vi "CMD Only (RT).vi"() -> ()   [LabVIEW 2013]
uses:
  Type Defs/Controller Names.ctl
  Type Defs/Sequence States.ctl
  Type Defs/CAN Mode.ctl
  Type Defs/Controller List.ctl
  <vilib>/FPGAPlugInAG/sbRIO-9626/niLvFpga_Open_sbRIO-9626.vi
  <vilib>/rvi/interface/common/dynamic/niFpgaDynamicAddResources.vi
  <vilib>/FPGAPlugInAG/Dynamic/niLvFpga_Reset_Dynamic.vi
  <vilib>/rvi/interface/common/niFpgaWaitOnOcc.vi
  <vilib>/Utility/error.llb/Error Cluster From Error Code.vi
  <vilib>/rvi/errors/niLvFpgaAdjustHostInterfaceError.vi
  <vilib>/FPGAPlugInAG/Dynamic/niLvFpga_Run_Dynamic.vi
  <vilib>/rvi/interface/nirviOpenFPGA/nirviOpenFPGA.xnode
  FPGA Bitfiles/CMD Only.lvbitx
  <vilib>/rvi/interface/nirviMethod/nirviMethod.xnode
  <vilib>/rvi/interface/nirviReadWriteControl/nirviReadWriteControl.xnode
  NiFpgaLv.dll
  <vilib>/rvi/interface/Simulation/niFpgaSimulationCallBeginRW.vi
  <vilib>/NI_Real-Time Target Support.lvlib
panel:
  in  "Monitoring Tab":enum32{"Page 1", "Page 2"}(tab)
  in  "Command":dbl min=10.0 max=100.0 step=0.1 format="%#.2f"
  in  "pb.Zero CMDs":bool
  out "CPU Usage:":dbl=7.74131899555212 format="%.1f"
  in  "Controller Type:":T1
  in  "Title":string="TI Automotive sbRIO, v2.1"
  out "CAN CMD":dbl
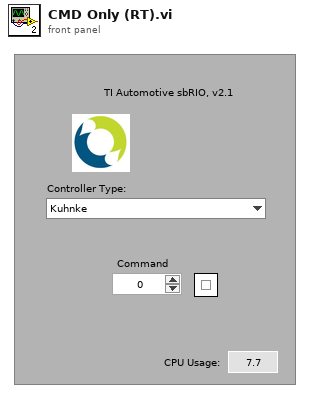
[diagram p1: front panel]
types:
  T1 = typedef "Controller Names.ctl" = enum16{"Kuhnke", "Conti", "Helbako", "TI PWM", "PSA", "Hella Gas", "Hella Diesel", "8 Comm", "10 Comm", "8 Comm Hella", "10 Comm Hella", "8 Comm Omron", "10 Comm Omron", "8 Comm Nissan", "10 Comm Nissan"}
  T2 = cluster{"Controller Name":T1, "CommSeg":i32, "PWM?":bool, "Frequency":i32, "Low Command":dbl, "High Command":dbl, "Stop Command":dbl, "Command Step":dbl, "Solenoid Stop?":bool, "Controller?":bool}
  T3 = typedef "CAN Mode.ctl" = enum16{"Init", "Read", "Write", "Close"}
  T4 = typedef "Sequence States.ctl" = enum16{"Main", "Init Files", "Init", "Save As", "Start Profile", "Check Step Time", "Restarts Alarm", "Run Step", "Stop Profile", "Cycle Reset", "Time Reset", "Time Reset All", "Time Set", "Tare CTs", "Save Profile", "Open Profile", "Get Profiles", "Update Screen", "Save Status", "Set Manual CMD", "Reset Restarts", "Reset Total Restarts", "Reset Cogs", "Disable Background", "Enable Background", "Get/Release Control", "Init AKLH", "Save AKLH", "Log Fuel Change", "Update Data Stream", "Init TenHz", "Read TenHz", "Remote Timer Reset", "Record Frequency Change", "Controller Change"}
  T5 = cluster{"Last Update":dbl, "Update Screen":bool, "Command":dbl, "Client?":bool, "Update Profile":bool, "Login":bool, "Stop Cmd":dbl, "Controller":cluster{"Controller Name":T1, "CommSeg":i32, "PWM?":bool, "Frequency":i32, "Low Command":dbl, "High Command":dbl, "Stop Command":dbl, "Command Step":dbl, "Solenoid Stop?":bool, "Controller?":bool}, "Controller Type:":T1}
  T6 = typedef "Controller List.ctl" = cluster{"Controller Name":T1, "CommSeg":i32, "PWM?":bool, "Frequency":i32, "Low Command":dbl, "High Command":dbl, "Stop Command":dbl, "Command Step":dbl, "Solenoid Stop?":bool, "Controller?":bool}[]
  T7 = typedef "LVRemotePanelConnectionsTypeDef.ctl" = cluster{"VI Name":string, "Remote":string, "UserName":string, "Port":i32, "Status":enum32{"Viewing", "Waiting For Control", "Controlling"}, "Create Time":timestamp, "Status Time":timestamp, "Control End Time":timestamp}[]
  T8 = typedef "NI_Real-Time Target Support.lvlib/RT CPU Load.ctl" = cluster{"Total (%)":dbl, "Time Critical (%)":dbl, "Timed Structures (%)":dbl, "High (%)":dbl, "Above Normal (%)":dbl, "Normal (%)":dbl, "Background (%)":dbl, "Idle (%)":dbl, "ISR (%)":dbl}
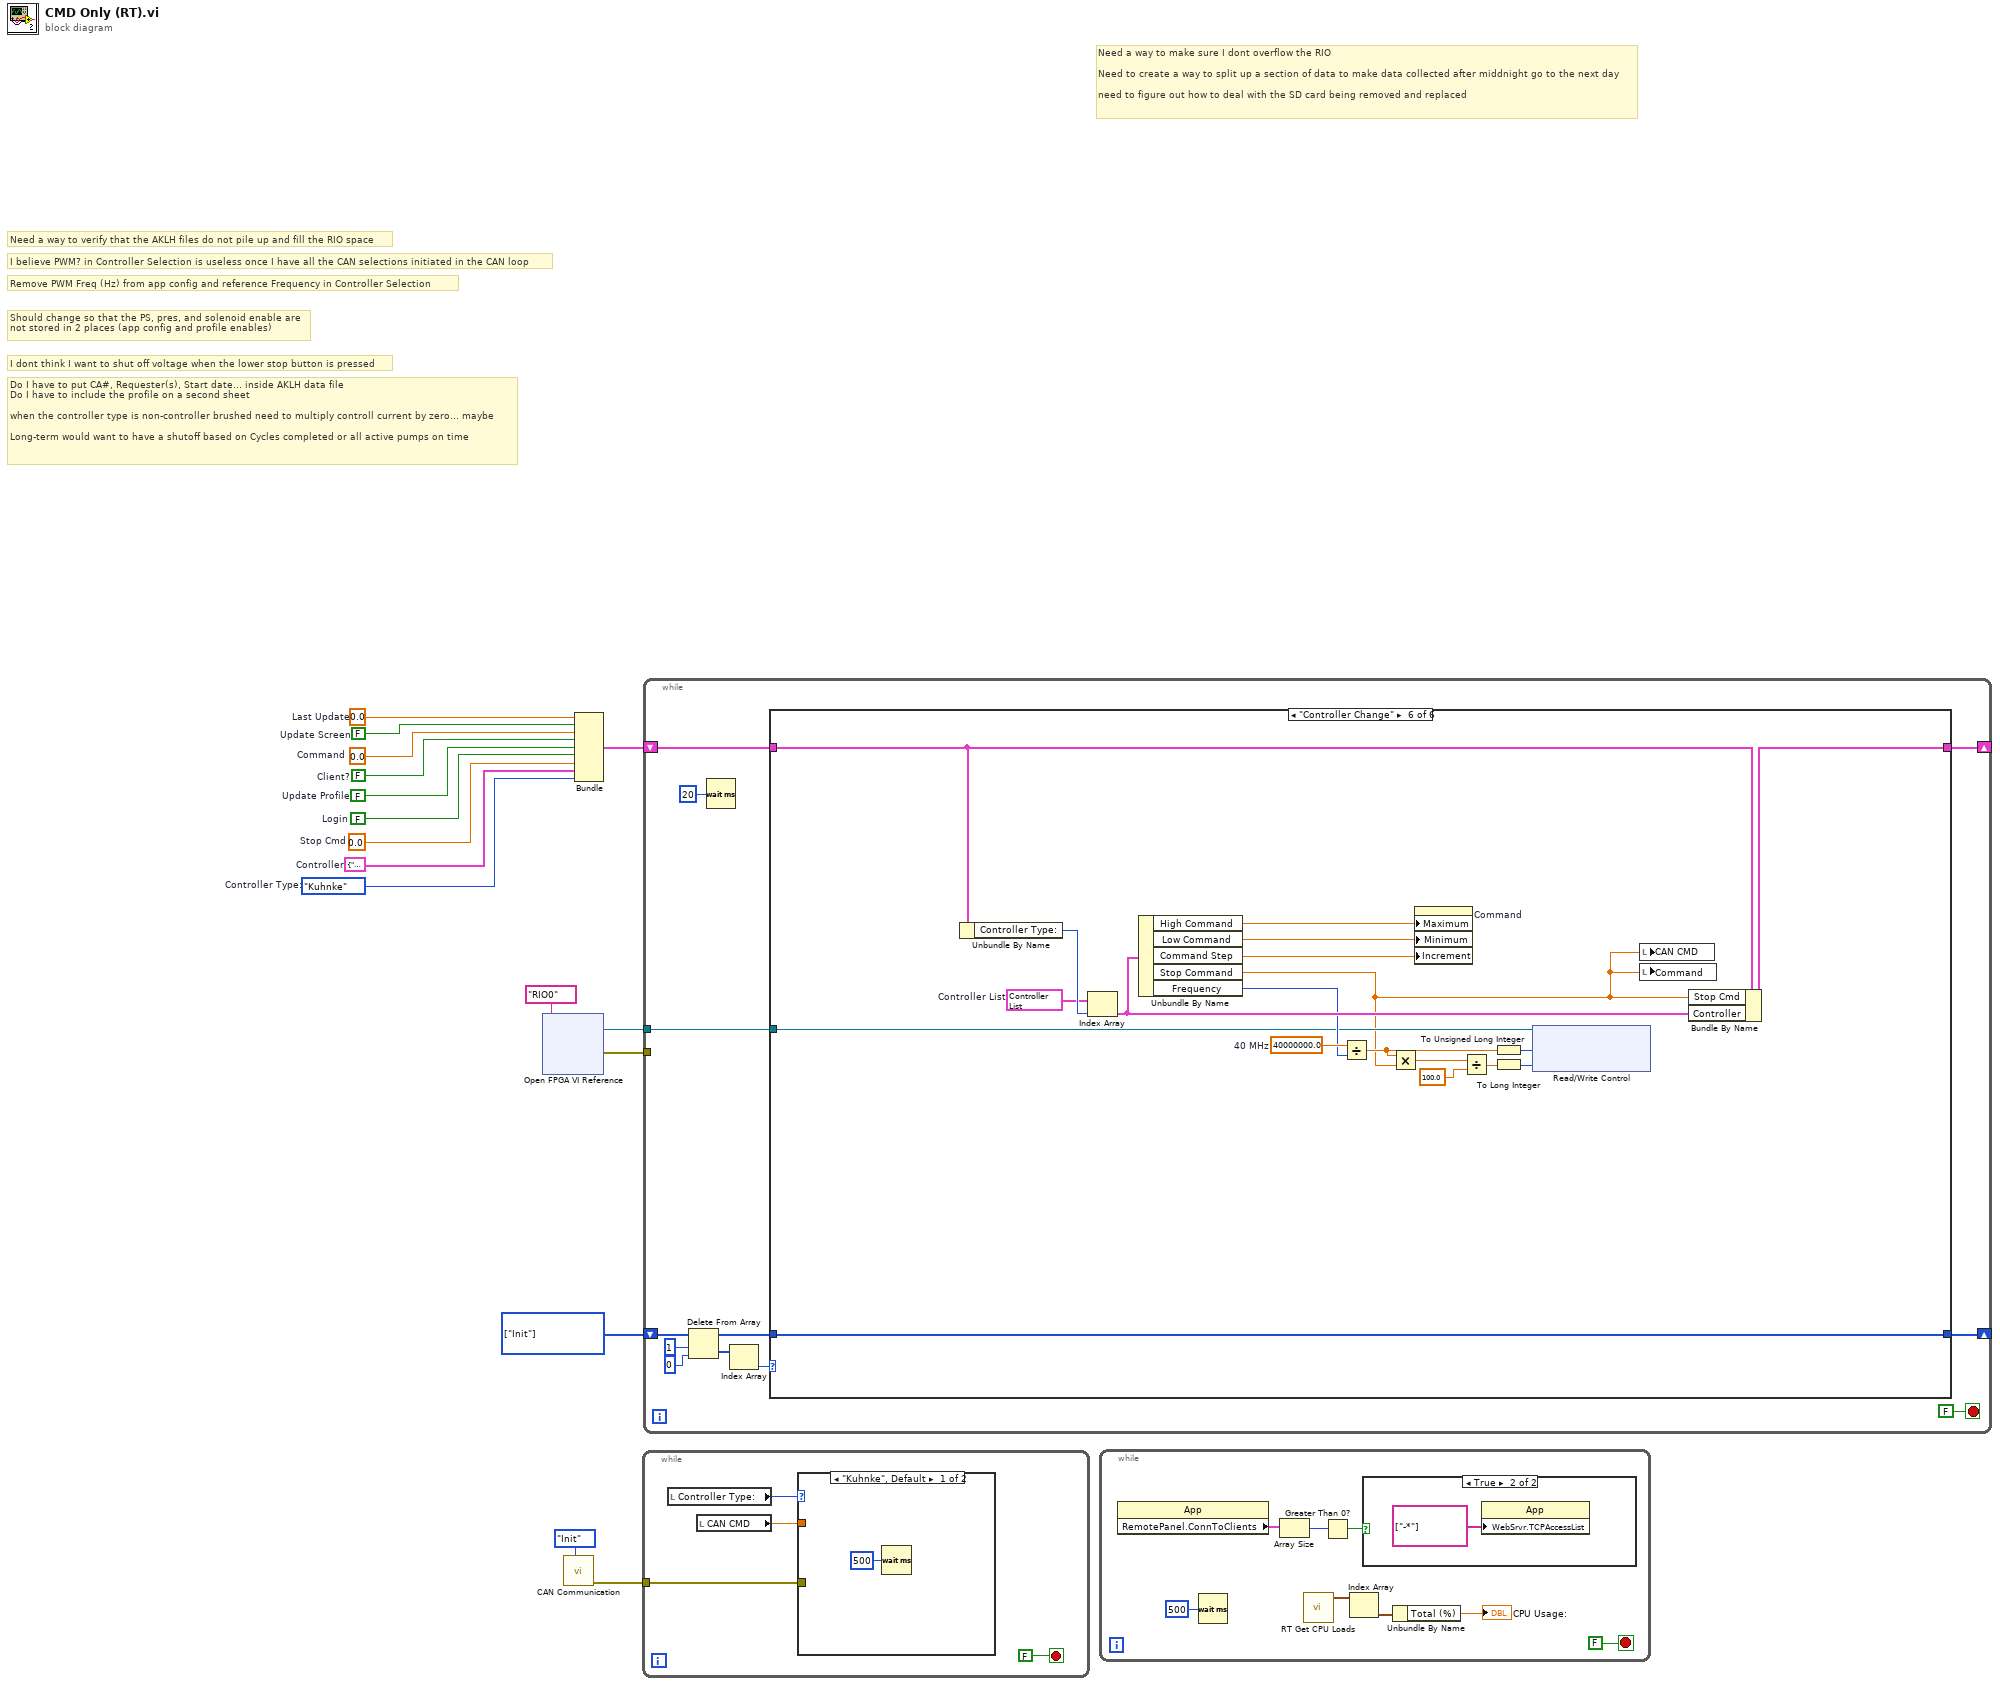
[diagram p0: block diagram]
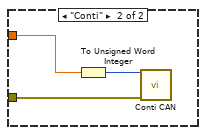
[diagram p2: hidden frame]
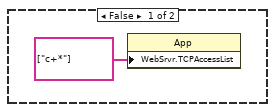
[diagram p3: hidden frame]
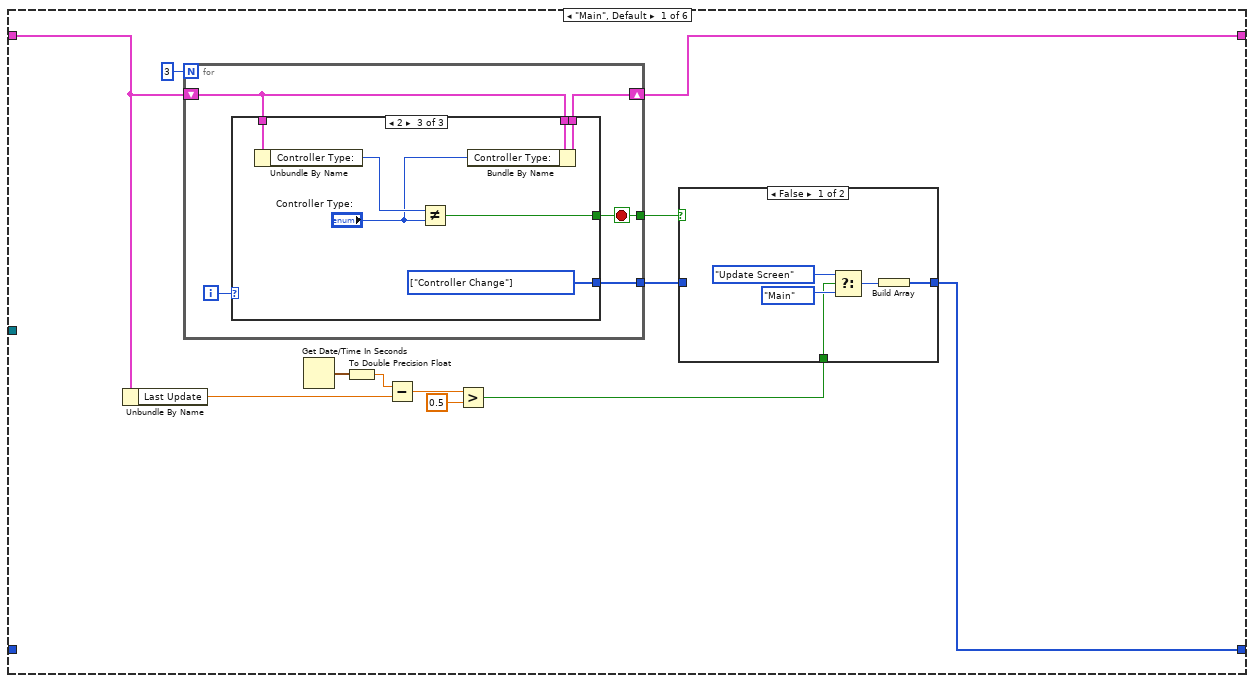
[diagram p4: hidden frame]
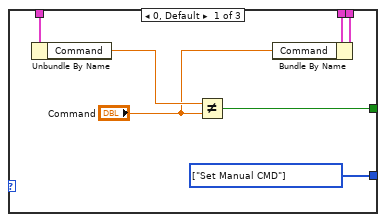
[diagram p5: hidden frame]
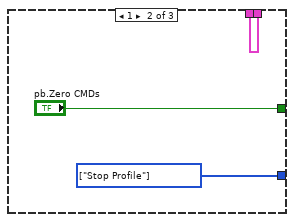
[diagram p6: hidden frame]
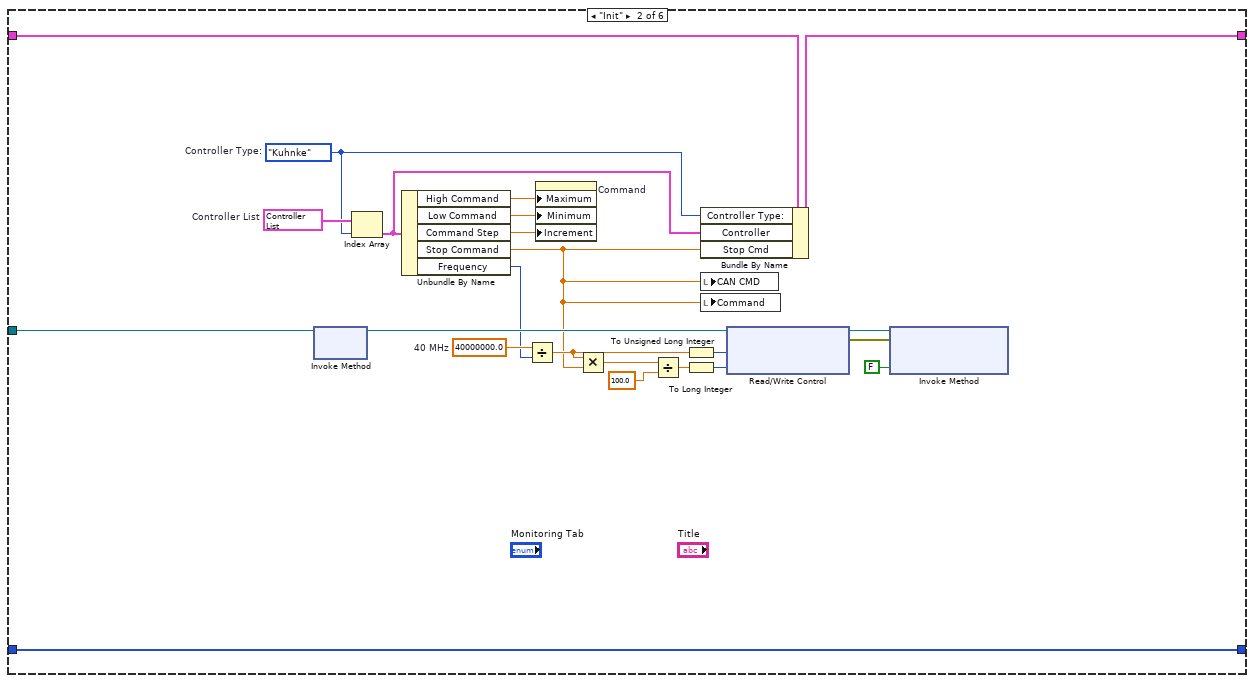
[diagram p8: hidden frame]
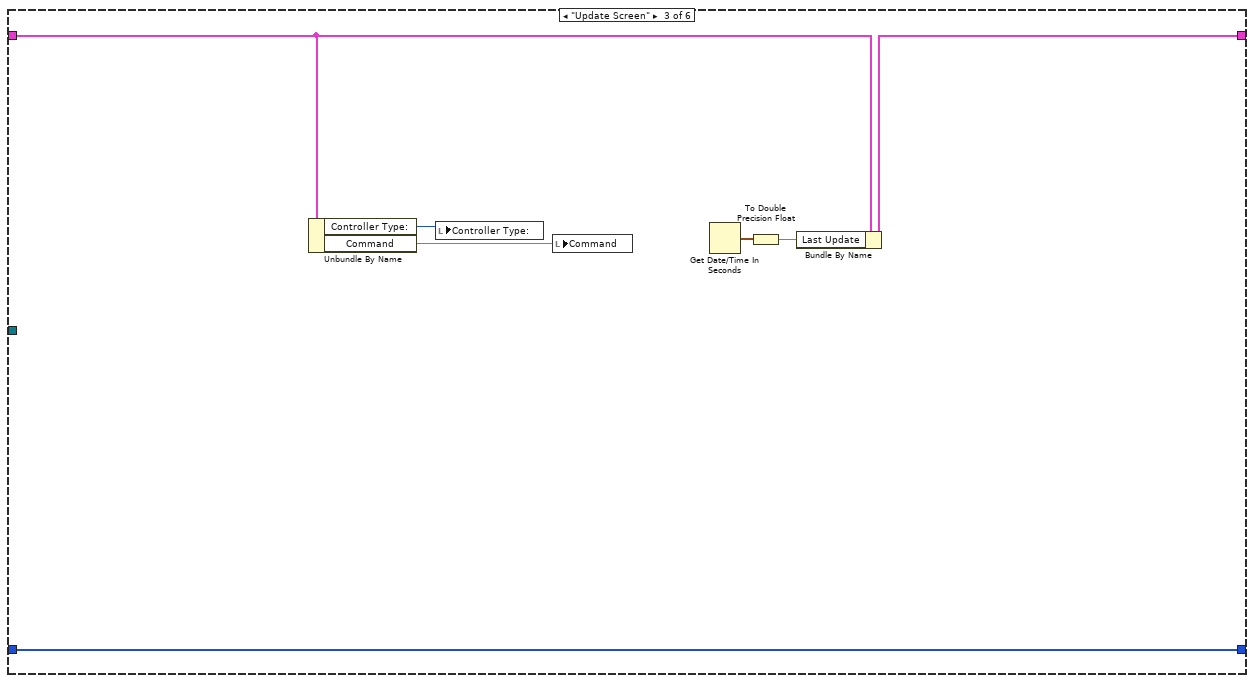
[diagram p9: hidden frame]
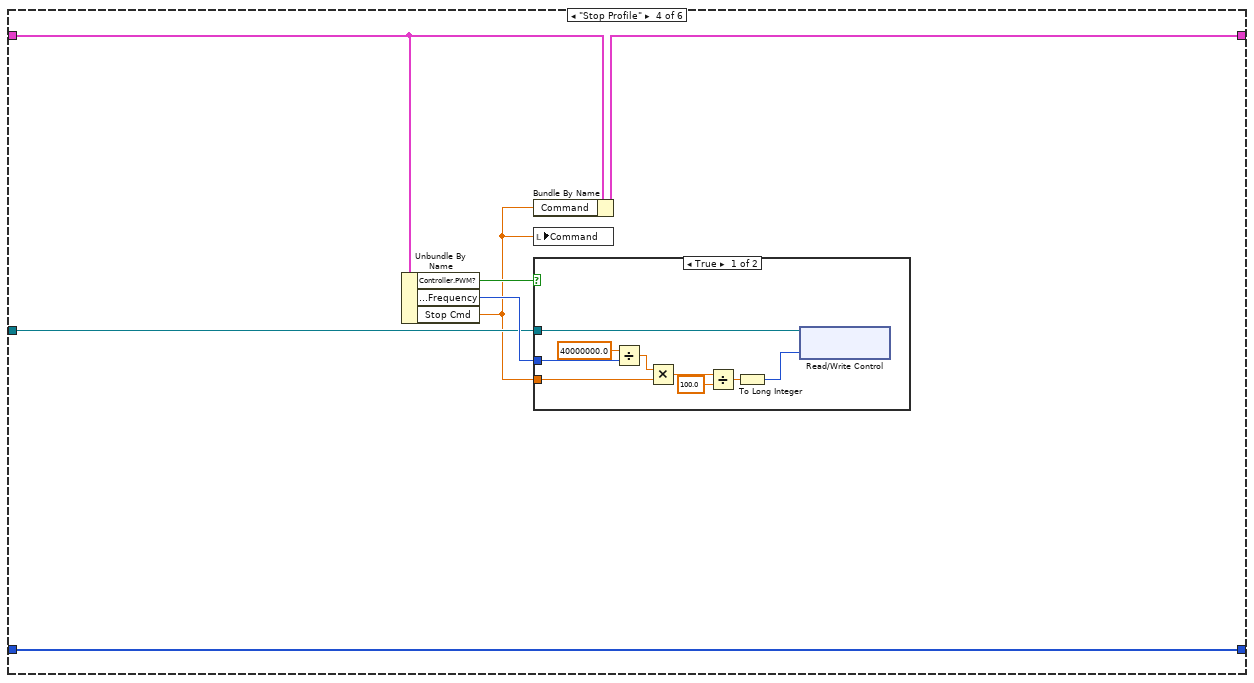
[diagram p10: hidden frame]
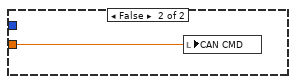
[diagram p11: hidden frame]
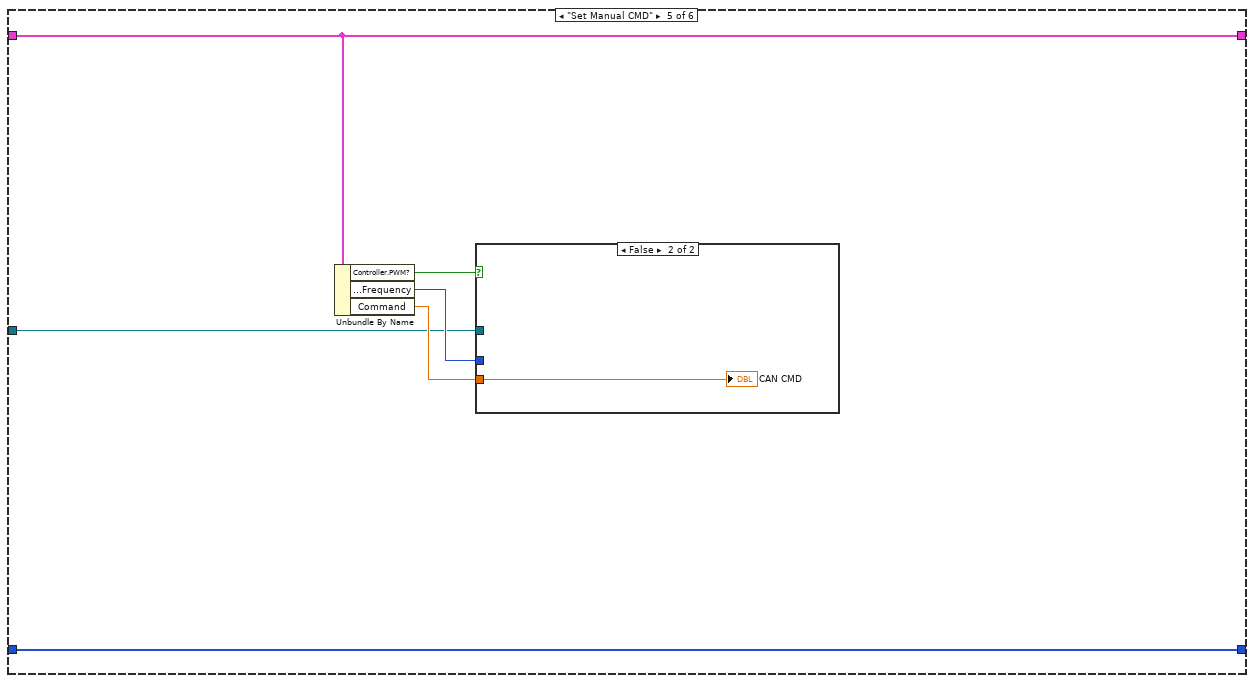
[diagram p12: hidden frame]
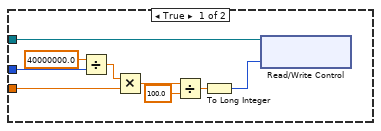
[diagram p13: hidden frame]
diagram:
  w1 = Controller_Names."Kuhnke"  # Controller Type:
  w2 = 0.0  # Command
  w3 = T2 {"Controller Name"=enum."Kuhnke", "CommSeg"=0, "PWM?"=FALSE, "Frequency"=0, "Low Command"=0.0, "High Command"=0.0, "Stop Command"=0.0, "Command Step"=0.0, "Solenoid Stop?"=FALSE, "Controller?"=FALSE}  # Controller
  w4 = 0.0  # Stop Cmd
  w15 = T4[] [enum."Init"] items=["Main", "Init Files", "Init", "Save As", "Start Profile", "Check Step Time", "Restarts Alarm", "Run Step", "Stop Profile", "Cycle Reset", "Time Reset", "Time Reset All", "Time Set", "Tare CTs", "Save Profile", "Open Profile", "Get Profiles", "Update Screen", "Save Status", "Set Manual CMD", "Reset Restarts", "Reset Total Restarts", "Reset Cogs", "Disable Background", "Enable Background", "Get/Release Control", "Init AKLH", "Save AKLH", "Log Fuel Change", "Update Data Stream", "Init TenHz", "Read TenHz", "Remote Timer Reset", "Record Frequency Change", "Controller Change"]
  w5 = FALSE  # Login
  w6 = FALSE  # Update Profile
  w7 = FALSE  # Client?
  w8 = FALSE  # Update Screen
  w9 = 0.0  # Last Update
  # "Need a way to make sure I dont overflow the RIO\n\nNeed to create a way to split up a section of data to make data collected after middnight go to the next day\n\nneed to figure out how to deal with the SD card being removed and replaced"
  # "Need a way to verify that the AKLH files do not pile up and fill the RIO space"
  # "I dont think I want to shut off voltage when the lower stop button is pressed"
  # "I believe PWM? in Controller Selection is useless once I have all the CAN selections initiated in the CAN loop"
  # "Remove PWM Freq (Hz) from app config and reference Frequency in Controller Selection"
  # "Do I have to put CA#, Requester(s), Start date... inside AKLH data file\nDo I have to include the profile on a second sheet\n\nwhen the controller type is non-controller brushed need to multiply controll current by zero... maybe\n\nLong-term would want to have a shutoff based on Cycles completed or all active pumps on time"
  # "Should change so that the PS, pres, and solenoid enable are\nnot stored in 2 places (app config and profile enables)"
  n1 = xnode "Open FPGA VI Reference"("resource name"=tag "RIO0") -> ("FPGA VI Reference Out"=w10:refnum<k20>, "error out"=w14:errorcluster)  [unwired: 1 in]
  n2 = call "CAN Communication.vi"("CAN Mode"=CAN_Mode."Init") -> ("Error OUT"=w12:errorcluster)  [unwired: 10 in]
  n3 = Bundle("Last Update"=w9, "Update Screen"=w8, "Command"=w2, "Client?"=w7, "Update Profile"=w6, "Login"=w5, "Stop Cmd"=w4, "Controller"=w3, "Controller Type:"=w1) -> (w16:T5)  [unwired: 1 in]
  n4 = while {
    tunnel: w12 -> [w19]
    stop <- FALSE stop-if-true
    n5 = local read "Controller Type:"() -> (w17:T1)
    n6 = local read "CAN CMD"() -> (w18:dbl)
    n7 = case shown="\"Kuhnke\", Default" w17 {
      tunnel: w19 -> [_ w24]
      tunnel: w18 -> [_ w23]
      frame "Kuhnke", Default {
        n8 = Wait (ms)(milliseconds to wait=u32 500) -> ()  [unwired: 1 out]
      }
      frame "Conti" {
        n9 = To Unsigned Word Integer(number=w23) -> (unsigned 16bit integer=w22:u16)
        n10 = call "Conti CAN.vi"("Error IN"=w24, "CMD"=w22) -> ()  [unwired: 9 in, 1 out]
      }
    }
  }
  n11 = while {
    shift-right: [w33] -> _
    shift-left: w15 -> [w31]
    shift-right: [w34] -> _
    shift-left: w16 -> [w35]
    tunnel: w10 -> [w32]
    tunnel: w14 -> [_]
    stop <- FALSE stop-if-true
    n12 = Delete From Array(array=w31, length=1, index=0 ("length")) -> (deleted portion=w27:T4[], array with subset deleted=w30:T4[])
    n13 = Wait (ms)(milliseconds to wait=u32 20) -> ()  [unwired: 1 out]
    n14 = Index Array(array=w27) -> (element=w26:T4)  [unwired: 1 in]
    n15 = case shown="\"Controller Change\"" w26 {
      tunnel: [w37 w92 w105 w113 w125 w154] -> w34
      tunnel: w35 -> [w47 w91 w106 w109 w125 w155]
      tunnel: [w38 w89 w103 w112 w126 w158] -> w33
      tunnel: w32 -> [_ w94 _ w108 w124 w141]
      tunnel: w30 -> [_ w89 w103 w112 w126 w158]
      frame "Main", Default {
        n16 = Unbundle By Name(w47) -> ("Last Update"=w48:dbl)
        n17 = for {
          N: 3 -> [_]
          shift-right: [w52] -> w37
          shift-left: w47 -> [w51]
          tunnel: [w50] -> w45
          tunnel: [w49] -> w46
          i -> [w53]
          stop <- w49 stop-if-true
          n18 = case shown="2" w53 {
            tunnel: w51 -> [w60 w62 w70]
            tunnel: [w59 w62 w69] -> w52
            tunnel: [w56 "pb.Zero CMDs" w66] -> w49
            tunnel: w51 -> [w58 _ w68]
            tunnel: [w55 w63 w65] -> w50
            frame 0, Default {
              w55 = T4[] [enum."Set Manual CMD"] items=["Main", "Init Files", "Init", "Save As", "Start Profile", "Check Step Time", "Restarts Alarm", "Run Step", "Stop Profile", "Cycle Reset", "Time Reset", "Time Reset All", "Time Set", "Tare CTs", "Save Profile", "Open Profile", "Get Profiles", "Update Screen", "Save Status", "Set Manual CMD", "Reset Restarts", "Reset Total Restarts", "Reset Cogs", "Disable Background", "Enable Background", "Get/Release Control", "Init AKLH", "Save AKLH", "Log Fuel Change", "Update Data Stream", "Init TenHz", "Read TenHz", "Remote Timer Reset", "Record Frequency Change", "Controller Change"]
              n19 = Unbundle By Name(w58) -> ("Command"=w57:dbl)
              n20 = Not Equal?(x=w57, y="Command") -> (x != y?=w56:bool)
              n21 = Bundle By Name(cluster=w60, "Command"="Command") -> (w59:T5)
            }
            frame 1 {
              w63 = T4[] [enum."Stop Profile"] items=["Main", "Init Files", "Init", "Save As", "Start Profile", "Check Step Time", "Restarts Alarm", "Run Step", "Stop Profile", "Cycle Reset", "Time Reset", "Time Reset All", "Time Set", "Tare CTs", "Save Profile", "Open Profile", "Get Profiles", "Update Screen", "Save Status", "Set Manual CMD", "Reset Restarts", "Reset Total Restarts", "Reset Cogs", "Disable Background", "Enable Background", "Get/Release Control", "Init AKLH", "Save AKLH", "Log Fuel Change", "Update Data Stream", "Init TenHz", "Read TenHz", "Remote Timer Reset", "Record Frequency Change", "Controller Change"]
            }
            frame 2 {
              w65 = T4[] [enum."Controller Change"] items=["Main", "Init Files", "Init", "Save As", "Start Profile", "Check Step Time", "Restarts Alarm", "Run Step", "Stop Profile", "Cycle Reset", "Time Reset", "Time Reset All", "Time Set", "Tare CTs", "Save Profile", "Open Profile", "Get Profiles", "Update Screen", "Save Status", "Set Manual CMD", "Reset Restarts", "Reset Total Restarts", "Reset Cogs", "Disable Background", "Enable Background", "Get/Release Control", "Init AKLH", "Save AKLH", "Log Fuel Change", "Update Data Stream", "Init TenHz", "Read TenHz", "Remote Timer Reset", "Record Frequency Change", "Controller Change"]
              n22 = Unbundle By Name(w68) -> ("Controller Type:"=w67:T1)
              n23 = Not Equal?(x=w67, y="Controller Type:") -> (x != y?=w66:bool)
              n24 = Bundle By Name(cluster=w70, "Controller Type:"="Controller Type:") -> (w69:T5)
            }
          }
        }
        n25 = Get Date/Time In Seconds() -> (seconds since 1Jan1904=w39:timestamp)
        n26 = To Double Precision Float(number=w39) -> (double precision float=w41:dbl)
        n27 = Subtract(x=w41, y=w48) -> (x-y=w42:dbl)
        n28 = Greater?(x=w42, y=0.5) -> (0:w44:bool)
        n29 = case shown="False" w46 {
          tunnel: [w71 w76] -> w38
          tunnel: w45 -> [_ w76]
          tunnel: w44 -> [w72 _]
          frame False {
            n30 = Select(t=Sequence_States."Update Screen", s=w72, f=Sequence_States."Main") -> (s? t:f=w73:T4)
            n31 = Build Array(w73) -> (w71:T4[])
          }
          frame True {
          }
        }
      }
      frame "Init" {
        w83 = Controller_Names."Kuhnke"  # Controller Type:
        w85 = T6 [{"Controller Name"=enum."Kuhnke", "CommSeg"=2, "PWM?"=TRUE, "Frequency"=100, "Low Command"=10.0, "High Command"=100.0, "Stop Command"=10.0, "Command Step"=0.1, "Solenoid Stop?"=FALSE, "Controller?"=FALSE}, {"Controller Name"=enum."Conti", "CommSeg"=2, "PWM?"=FALSE, "Frequency"=100, "Low Command"=0.0, "High Command"=800.0, "Stop Command"=0.0, "Command Step"=1.0, "Solenoid Stop?"=FALSE, "Controller?"=FALSE}, {"Controller Name"=enum."Helbako", "CommSeg"=2, "PWM?"=FALSE, "Frequency"=100, "Low Command"=0.0, "High Command"=100.0, "Stop Command"=0.0, "Command Step"=0.1, "Solenoid Stop?"=FALSE, "Controller?"=FALSE}, {"Controller Name"=enum."TI PWM", "CommSeg"=2, "PWM?"=TRUE, "Frequency"=100, "Low Command"=0.0, "High Command"=100.0, "Stop Command"=0.0, "Command Step"=0.1, "Solenoid Stop?"=FALSE, "Controller?"=FALSE}, {"Controller Name"=enum."PSA", "CommSeg"=2, "PWM?"=TRUE, "Frequency"=100, "Low Command"=5.0, "High Command"=95.0, "Stop Command"=5.0, "Command Step"=0.1, "Solenoid Stop?"=FALSE, "Controller?"=FALSE}, {"Controller Name"=enum."Hella Gas", "CommSeg"=2, "PWM?"=FALSE, "Frequency"=100, "Low Command"=0.0, "High Command"=800.0, "Stop Command"=0.0, "Command Step"=1.0, "Solenoid Stop?"=TRUE, "Controller?"=FALSE}, {"Controller Name"=enum."Hella Diesel", "CommSeg"=2, "PWM?"=FALSE, "Frequency"=100, "Low Command"=370.0, "High Command"=461.0, "Stop Command"=370.0, "Command Step"=1.0, "Solenoid Stop?"=TRUE, "Controller?"=FALSE}, {"Controller Name"=enum."8 Comm", "CommSeg"=8, "PWM?"=FALSE, "Frequency"=100, "Low Command"=0.0, "High Command"=1.0, "Stop Command"=0.0, "Command Step"=1.0, "Solenoid Stop?"=FALSE, "Controller?"=FALSE}, {"Controller Name"=enum."10 Comm", "CommSeg"=10, "PWM?"=FALSE, "Frequency"=100, "Low Command"=0.0, "High Command"=1.0, "Stop Command"=0.0, "Command Step"=1.0, "Solenoid Stop?"=FALSE, "Controller?"=FALSE}, {"Controller Name"=enum."8 Comm Hella", "CommSeg"=8, "PWM?"=TRUE, "Frequency"=150, "Low Command"=0.0, "High Command"=50.0, "Stop Command"=80.0, "Command Step"=0.1, "Solenoid Stop?"=FALSE, "Controller?"=FALSE}, {"Controller Name"=enum."10 Comm Hella", "CommSeg"=10, "PWM?"=TRUE, "Frequency"=150, "Low Command"=0.0, "High Command"=50.0, "Stop Command"=80.0, "Command Step"=0.1, "Solenoid Stop?"=FALSE, "Controller?"=FALSE}, {"Controller Name"=enum."8 Comm Omron", "CommSeg"=8, "PWM?"=TRUE, "Frequency"=150, "Low Command"=5.0, "High Command"=50.0, "Stop Command"=75.0, "Command Step"=0.1, "Solenoid Stop?"=FALSE, "Controller?"=FALSE}, {"Controller Name"=enum."10 Comm Omron", "CommSeg"=10, "PWM?"=TRUE, "Frequency"=150, "Low Command"=5.0, "High Command"=50.0, "Stop Command"=75.0, "Command Step"=0.1, "Solenoid Stop?"=FALSE, "Controller?"=FALSE}, {"Controller Name"=enum."8 Comm Nissan", "CommSeg"=8, "PWM?"=TRUE, "Frequency"=10, "Low Command"=50.0, "High Command"=90.0, "Stop Command"=50.0, "Command Step"=0.1, "Solenoid Stop?"=TRUE, "Controller?"=FALSE}, {"Controller Name"=enum."10 Comm Nissan", "CommSeg"=10, "PWM?"=TRUE, "Frequency"=10, "Low Command"=50.0, "High Command"=90.0, "Stop Command"=50.0, "Command Step"=0.1, "Solenoid Stop?"=TRUE, "Controller?"=FALSE}]  # Controller List
        w95 = 40000000.0  # 40 MHz
        n32 = xnode "Invoke Method"("FPGA VI Reference In"=w94) -> ("FPGA VI Reference Out"=w93:refnum<k20>)  [unwired: 1 in, 1 out]
        n33 = Index Array(array=w85, index=w83) -> (element=w84:T2)
        n34 = Unbundle By Name(w84) -> ("High Command"=w88:dbl, "Low Command"=w87:dbl, "Command Step"=w86:dbl, "Stop Command"=w80:dbl, "Frequency"=w90:i32)
        n35 = Divide(x=w95, y=w90) -> (x/y=w81:dbl)
        n36 = property on="Command" class="DigNum (strict)"("Maximum"=w88, "Minimum"=w87, "Increment"=w86) -> ()  [unwired: 2 in, 2 out]
        n37 = Multiply(x=w81, y=w80) -> (x*y=w78:dbl)
        n38 = Divide(x=w78, y=100.0 ("x")) -> (x/y=w82:dbl)
        n39 = To Unsigned Long Integer(number=w81) -> (unsigned 32bit integer=w99:u32)
        n40 = To Long Integer(number=w82) -> (32bit integer=w79:i32)
        n41 = Bundle By Name(cluster=w91, "Controller Type:"=w83, "Controller"=w84, "Stop Cmd"=w80) -> (w92:T5)
        n42 = local write "CAN CMD"(w80) -> ()
        n43 = local write "Command"(w80) -> ()
        n44 = xnode "Read/Write Control"("FPGA VI Reference In"=w93, "PWM Period (Ticks)"=w99, "Duty (Ticks) 1"=w79) -> ("FPGA VI Reference Out"=w97:refnum<k20>, "error out"=w96:errorcluster)  [unwired: 1 in]
        n45 = xnode "Invoke Method"("FPGA VI Reference In"=w97, "error in"=w96, "Wait Until Done (F)"=FALSE) -> ()  [unwired: 2 out]
      }
      frame "Update Screen" {
        n46 = Unbundle By Name(w106) -> ("Controller Type:"=w104:T1, "Command"=w102:dbl)
        n47 = local write "Controller Type:"(w104) -> ()
        n48 = local write "Command"(w102) -> ()
        n49 = Get Date/Time In Seconds() -> (seconds since 1Jan1904=w101:timestamp)
        n50 = To Double Precision Float(number=w101) -> (double precision float=w100:dbl)
        n51 = Bundle By Name(cluster=w106, "Last Update"=w100) -> (w105:T5)
      }
      frame "Stop Profile" {
        n52 = Unbundle By Name(w109) -> ("Controller.PWM?"=w110:bool, "Controller.Frequency"=w111:i32, "Stop Cmd"=w107:dbl)
        n53 = Bundle By Name(cluster=w109, "Command"=w107) -> (w113:T5)
        n54 = local write "Command"(w107) -> ()
        n55 = case shown="True" w110 {
          tunnel: w108 -> [w122 _]
          tunnel: w111 -> [w115 _]
          tunnel: w107 -> [w121 w123]
          frame True {
            n56 = Divide(x=40000000.0 ("40 MHz"), y=w115) -> (x/y=w120:dbl)
            n57 = Multiply(x=w120, y=w121) -> (x*y=w116:dbl)
            n58 = Divide(x=w116, y=100.0 ("%")) -> (x/y=w118:dbl)
            n59 = To Long Integer(number=w118) -> (32bit integer=w114:i32)
            n60 = xnode "Read/Write Control"("FPGA VI Reference In"=w122, "Duty (Ticks) 1"=w114) -> ()  [unwired: 1 in, 2 out]
          }
          frame False {
            n61 = local write "CAN CMD"(w123) -> ()
          }
        }
      }
      frame "Set Manual CMD" {
        n62 = Unbundle By Name(w125) -> ("Controller.PWM?"=w128:bool, "Controller.Frequency"=w129:i32, "Command"=w127:dbl)
        n63 = case shown="False" w128 {
          tunnel: w124 -> [w138 _]
          tunnel: w129 -> [w131 _]
          tunnel: w127 -> [w137 w139]
          frame True {
            n64 = Divide(x=40000000.0 ("40 MHz"), y=w131) -> (x/y=w136:dbl)
            n65 = Multiply(x=w136, y=w137) -> (x*y=w132:dbl)
            n66 = Divide(x=w132, y=100.0 ("%")) -> (x/y=w134:dbl)
            n67 = To Long Integer(number=w134) -> (32bit integer=w130:i32)
            n68 = xnode "Read/Write Control"("FPGA VI Reference In"=w138, "Duty (Ticks) 1"=w130) -> ()  [unwired: 1 in, 2 out]
          }
          frame False {
            "CAN CMD" <- w139
          }
        }
      }
      frame "Controller Change" {
        w148 = 40000000.0  # 40 MHz
        w156 = T6 [{"Controller Name"=enum."Kuhnke", "CommSeg"=2, "PWM?"=TRUE, "Frequency"=100, "Low Command"=10.0, "High Command"=100.0, "Stop Command"=10.0, "Command Step"=0.1, "Solenoid Stop?"=FALSE, "Controller?"=FALSE}, {"Controller Name"=enum."Conti", "CommSeg"=2, "PWM?"=FALSE, "Frequency"=100, "Low Command"=0.0, "High Command"=800.0, "Stop Command"=0.0, "Command Step"=1.0, "Solenoid Stop?"=FALSE, "Controller?"=FALSE}, {"Controller Name"=enum."Helbako", "CommSeg"=2, "PWM?"=FALSE, "Frequency"=100, "Low Command"=0.0, "High Command"=100.0, "Stop Command"=0.0, "Command Step"=0.1, "Solenoid Stop?"=FALSE, "Controller?"=FALSE}, {"Controller Name"=enum."TI PWM", "CommSeg"=2, "PWM?"=TRUE, "Frequency"=100, "Low Command"=0.0, "High Command"=100.0, "Stop Command"=0.0, "Command Step"=0.1, "Solenoid Stop?"=FALSE, "Controller?"=FALSE}, {"Controller Name"=enum."PSA", "CommSeg"=2, "PWM?"=TRUE, "Frequency"=100, "Low Command"=5.0, "High Command"=95.0, "Stop Command"=5.0, "Command Step"=0.1, "Solenoid Stop?"=FALSE, "Controller?"=FALSE}, {"Controller Name"=enum."Hella Gas", "CommSeg"=2, "PWM?"=FALSE, "Frequency"=100, "Low Command"=0.0, "High Command"=800.0, "Stop Command"=0.0, "Command Step"=1.0, "Solenoid Stop?"=TRUE, "Controller?"=FALSE}, {"Controller Name"=enum."Hella Diesel", "CommSeg"=2, "PWM?"=FALSE, "Frequency"=100, "Low Command"=370.0, "High Command"=461.0, "Stop Command"=370.0, "Command Step"=1.0, "Solenoid Stop?"=TRUE, "Controller?"=FALSE}, {"Controller Name"=enum."8 Comm", "CommSeg"=8, "PWM?"=FALSE, "Frequency"=100, "Low Command"=0.0, "High Command"=1.0, "Stop Command"=0.0, "Command Step"=1.0, "Solenoid Stop?"=FALSE, "Controller?"=FALSE}, {"Controller Name"=enum."10 Comm", "CommSeg"=10, "PWM?"=FALSE, "Frequency"=100, "Low Command"=0.0, "High Command"=1.0, "Stop Command"=0.0, "Command Step"=1.0, "Solenoid Stop?"=FALSE, "Controller?"=FALSE}, {"Controller Name"=enum."8 Comm Hella", "CommSeg"=8, "PWM?"=TRUE, "Frequency"=150, "Low Command"=0.0, "High Command"=50.0, "Stop Command"=80.0, "Command Step"=0.1, "Solenoid Stop?"=FALSE, "Controller?"=FALSE}, {"Controller Name"=enum."10 Comm Hella", "CommSeg"=10, "PWM?"=TRUE, "Frequency"=150, "Low Command"=0.0, "High Command"=50.0, "Stop Command"=80.0, "Command Step"=0.1, "Solenoid Stop?"=FALSE, "Controller?"=FALSE}, {"Controller Name"=enum."8 Comm Omron", "CommSeg"=8, "PWM?"=TRUE, "Frequency"=150, "Low Command"=5.0, "High Command"=50.0, "Stop Command"=75.0, "Command Step"=0.1, "Solenoid Stop?"=FALSE, "Controller?"=FALSE}, {"Controller Name"=enum."10 Comm Omron", "CommSeg"=10, "PWM?"=TRUE, "Frequency"=150, "Low Command"=5.0, "High Command"=50.0, "Stop Command"=75.0, "Command Step"=0.1, "Solenoid Stop?"=FALSE, "Controller?"=FALSE}, {"Controller Name"=enum."8 Comm Nissan", "CommSeg"=8, "PWM?"=TRUE, "Frequency"=10, "Low Command"=50.0, "High Command"=90.0, "Stop Command"=50.0, "Command Step"=0.1, "Solenoid Stop?"=TRUE, "Controller?"=FALSE}, {"Controller Name"=enum."10 Comm Nissan", "CommSeg"=10, "PWM?"=TRUE, "Frequency"=10, "Low Command"=50.0, "High Command"=90.0, "Stop Command"=50.0, "Command Step"=0.1, "Solenoid Stop?"=TRUE, "Controller?"=FALSE}]  # Controller List
        n69 = Unbundle By Name(w155) -> ("Controller Type:"=w157:T1)
        n70 = Index Array(array=w156, index=w157) -> (element=w153:T2)
        n71 = Unbundle By Name(w153) -> ("High Command"=w152:dbl, "Low Command"=w151:dbl, "Command Step"=w150:dbl, "Stop Command"=w140:dbl, "Frequency"=w142:i32)
        n72 = Divide(x=w148, y=w142) -> (x/y=w146:dbl)
        n73 = Multiply(x=w146, y=w140) -> (x*y=w144:dbl)
        n74 = property on="Command" class="DigNum (strict)"("Maximum"=w152, "Minimum"=w151, "Increment"=w150) -> ()  [unwired: 2 in, 2 out]
        n75 = Divide(x=w144, y=100.0 ("x")) -> (x/y=w147:dbl)
        n76 = To Unsigned Long Integer(number=w146) -> (unsigned 32bit integer=w149:u32)
        n77 = To Long Integer(number=w147) -> (32bit integer=w145:i32)
        n78 = xnode "Read/Write Control"("FPGA VI Reference In"=w141, "PWM Period (Ticks)"=w149, "Duty (Ticks) 1"=w145) -> ()  [unwired: 1 in, 2 out]
        n79 = local write "CAN CMD"(w140) -> ()
        n80 = local write "Command"(w140) -> ()
        n81 = Bundle By Name(cluster=w155, "Stop Cmd"=w140, "Controller"=w153) -> (w154:T5)
      }
    }
  }
  n82 = while {
    stop <- FALSE stop-if-true
    n83 = property class="App"() -> ("RemotePanel.ConnToClients"=w163:T7)  [unwired: 2 in, 2 out]
    n84 = Wait (ms)(milliseconds to wait=u32 500) -> ()  [unwired: 1 out]
    n85 = Array Size(array=w163) -> (size(s)=w164:i32)
    n86 = call <vilib>:"RT Get CPU Loads.vi"() -> ("CPU loads"=w160:T8[])  [unwired: 10 in, 1 out]
    n87 = Greater Than 0?(x=w164) -> (x > 0?=w162:bool)
    n88 = Index Array(array=w160) -> (element=w161:T8)  [unwired: 1 in]
    n89 = case shown="True" w162 {
      frame False {
        n90 = property class="App"("WebSrvr.TCPAccessList"=string[] ["c+*"] ("Web Server:TCP/IP Access List")) -> ()  [unwired: 2 in, 2 out]
      }
      frame True {
        n91 = property class="App"("WebSrvr.TCPAccessList"=string[] ["-*"] ("Web Server:TCP/IP Access List")) -> ()  [unwired: 2 in, 2 out]
      }
    }
    n92 = Unbundle By Name(w161) -> ("Total (%)"=→"CPU Usage:":dbl)
  }
